vi "match_labview_version.vi"() -> ()   [LabVIEW 2021]
uses:
  <vilib>/regexp/Match Regular Expression.xnode
panel:
  out "versions":string[](array[string])
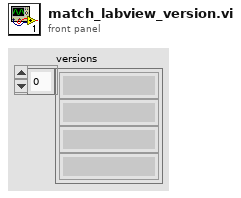
[diagram p1: front panel]
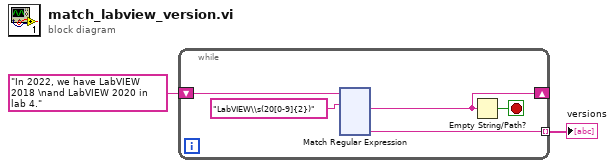
[diagram p0: block diagram]
diagram:
  n1 = while {
    shift-right: [w5] -> _
    shift-left: "In 2022, we have LabVIEW 2018 \nand LabVIEW 2020 in lab 4." ("input string") -> [w7]
    tunnel: [w3] -> w1 mode=indexing
    stop <- w4 stop-if-true
    n2 = xnode "Match Regular Expression"("input string"=w7, "regular expression"="LabVIEW\\s(20[0-9]{2})") -> ("after match"=w5:string, "submatch 1"=w3:string)  [unwired: 4 in, 4 out]
    n3 = Empty String/Path?(string/path=w5) -> (empty?=w4:bool)
  }
  "versions" <- w1
